vi "startIVSweepAndWait.vi"(8 "error in (no error)":errorcluster, 10 "Configure Sweep":T1 {"Sweep End (V)" format="%#_6p"; "Sweep Start (V)" format="%#_6p"; "Initial Wait (s)" format="%#_6p"}, 11 "Instrument.Lockin in":refnum<class "Instrument.Lockin.lvclass">) -> (0 "error out":errorcluster, 3 "Instrument.Lockin out":refnum<class "Instrument.Lockin.lvclass">)   [LabVIEW 2016, in "Instrument.Lockin.lvclass"]
uses:
  Instrument.Lockin.lvclass
  Lockin.DAQ/Typedefs/Sweep Configuration--Cluster.ctl
  Lockin.DAQ/Typedefs/Sweep Pattern--Enum.ctl
  Lockin.DAQ/Lockin.DAQ.lvclass
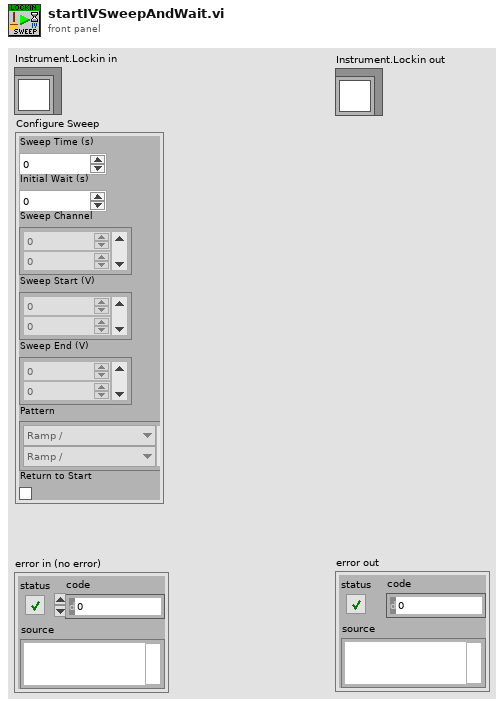
[diagram p1: front panel]
types:
  T1 = typedef "Lockin.DAQ.lvclass/Sweep Configuration--Cluster.ctl" = cluster{"Sweep Time (s)":dbl, "Initial Wait (s)":dbl, "Sweep Channel":i32[], "Sweep Start (V)":dbl[], "Sweep End (V)":dbl[], "Pattern":T2[], "Return to Start":bool}
  T2 = typedef "Lockin.DAQ.lvclass/Sweep Pattern--Enum.ctl" = enum16{"Ramp /", "Ramp /\\", "Smooth Ramp _/", "Smooth Ramp _/\\_", "Frequency"}
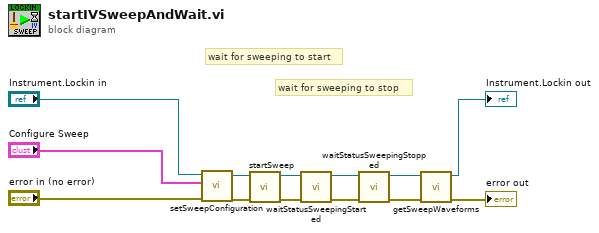
[diagram p0: block diagram]
diagram:
  # "wait for sweeping to stop"
  # "wait for sweeping to start"
  n1 = call "setSweepConfiguration.vi"("error in (no error)"="error in (no error)", "Configure Sweep"="Configure Sweep", "Instrument.Lockin in"="Instrument.Lockin in") -> ("error out"=w9:errorcluster, "Instrument.Lockin out"=w10:refnum<class "Instrument.Lockin.lvclass">)  [unwired: 7 in]
  n2 = call "startSweep.vi"("error in (no error)"=w9, "Instrument.Lockin in"=w10) -> ("error out"=w5:errorcluster, "Instrument.Lockin out"=w6:refnum<class "Instrument.Lockin.lvclass">)  [unwired: 8 in]
  n3 = call "waitStatusSweepingStarted.vi"("error in (no error)"=w5, "Instrument.Lockin in"=w6) -> ("error out"=w4:errorcluster, "Instrument.Lockin out"=w7:refnum<class "Instrument.Lockin.lvclass">)  [unwired: 8 in]
  n4 = call "waitStatusSweepingStopped.vi"("error in (no error)"=w4, "Instrument.Lockin in"=w7) -> ("error out"=w3:errorcluster, "Instrument.Lockin out"=w2:refnum<class "Instrument.Lockin.lvclass">)  [unwired: 8 in]
  n5 = call "getSweepWaveforms.vi"("error in (no error)"=w3, "Instrument.Lockin in"=w2) -> ("error out"=→"error out":errorcluster, "Instrument.Lockin out"=→"Instrument.Lockin out":refnum<class "Instrument.Lockin.lvclass">)  [unwired: 6 in, 2 out]
